vi "7.3-SelectYourBehaviorEventHandler.vi"(0 "NewVal":T1(ring), 1 "Controls[]":refnum<vi>[](array[refnum]), 2 "Select Pen Attributes":T2) -> ()   [LabVIEW 2010]
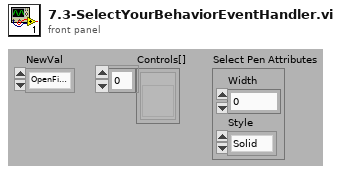
[diagram p1: front panel]
types:
  T1 = enum16{"OpenFieldTransit", "WallFollow", "LaneFollow", "ManualMode"}
  T2 = cluster{"Width":u16, "Style":enum32{"Solid", "Dash", "Dot", "DashDot", "DashDotDot"}}
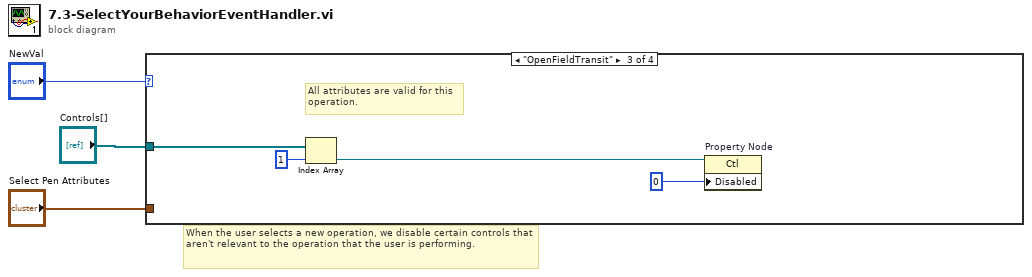
[diagram p0: block diagram]
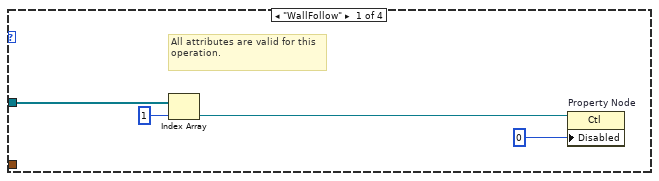
[diagram p2: hidden frame]
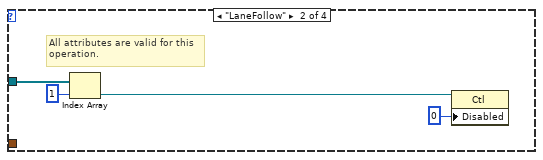
[diagram p3: hidden frame]
diagram:
  # "When the user selects a new operation, we disable certain controls that aren't relevant to the operation that the user is performing."
  n1 = case shown="\"OpenFieldTransit\"" "NewVal" {
    tunnel: "Controls[]" -> [w7 w8 w12 _]
    tunnel: "Select Pen Attributes" -> [_ _ _ _]
    frame "WallFollow" {
      # "All attributes are valid for this\noperation."
      n2 = Index Array "Index Array"(array=w7, index=1) -> (element=w5:refnum<vi>)
      n3 = property on="Property Node" class="Ctl"(reference=w5, "Disabled"=u8 0) -> ()  [unwired: 1 in, 2 out]
    }
    frame "LaneFollow" {
      # "All attributes are valid for this\noperation."
      n4 = Index Array(array=w8, index=1) -> (element=w10:refnum<vi>)
      n5 = property class="Ctl"(reference=w10, "Disabled"=u8 0) -> ()  [unwired: 1 in, 2 out]
    }
    frame "OpenFieldTransit" {
      # "All attributes are valid for this\noperation."
      n6 = Index Array "Index Array"(array=w12, index=1) -> (element=w14:refnum<vi>)
      n7 = property on="Property Node" class="Ctl"(reference=w14, "Disabled"=u8 0) -> ()  [unwired: 1 in, 2 out]
    }
    frame "ManualMode" {
    }
  }
